vi "Write Waveform Data.vi"(8 "error in (no error)":errorcluster, 10 "Waveform Data":waveform(dbl), 11 "Composite Waveform in":refnum<class "Composite Waveform.lvclass">) -> (0 "error out":errorcluster, 3 "Composite Waveform out":refnum<class "Composite Waveform.lvclass">)   [LabVIEW 2020, in "Composite Waveform.lvclass"]
uses:
  Composite Waveform.lvclass
  Analog Waveform/Analog Waveform.lvclass
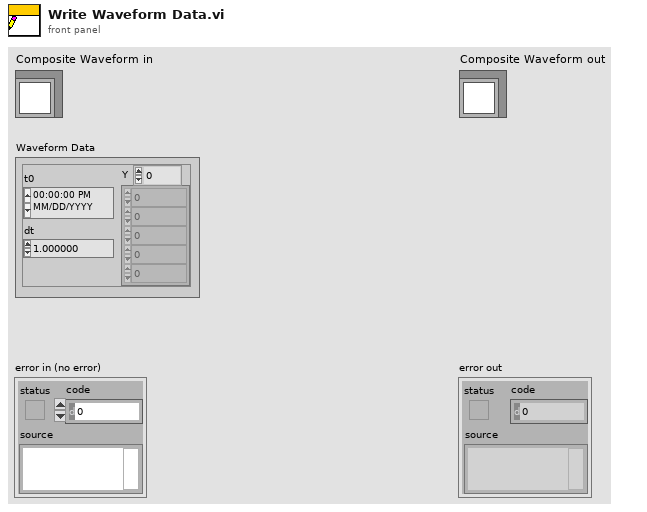
[diagram p1: front panel]
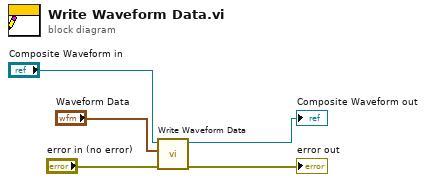
[diagram p0: block diagram]
diagram:
  n1 = call-parent "Write Waveform Data.vi"("error in (no error)"="error in (no error)", "Waveform Data"="Waveform Data", "Analog Waveform in"="Composite Waveform in") -> ("error out"=→"error out":errorcluster, "Analog Waveform out"=→"Composite Waveform out":refnum<class "Composite Waveform.lvclass">)  [unwired: 7 in]
